vi "Toggle Allow Undefined Strings.vi"(8 "error in (no error)":errorcluster, 10 "Allow Undefined Strings":bool, 11 "List Data Type in":refnum<class "List Data Type.lvclass">) -> (0 "error out":errorcluster, 3 "List Data Type out":refnum<class "List Data Type.lvclass">)   [LabVIEW 2018, in "List Data Type.lvclass"]
uses:
  List Data Type.lvclass
  List Data Type.lvclass/List Data Type.ctl
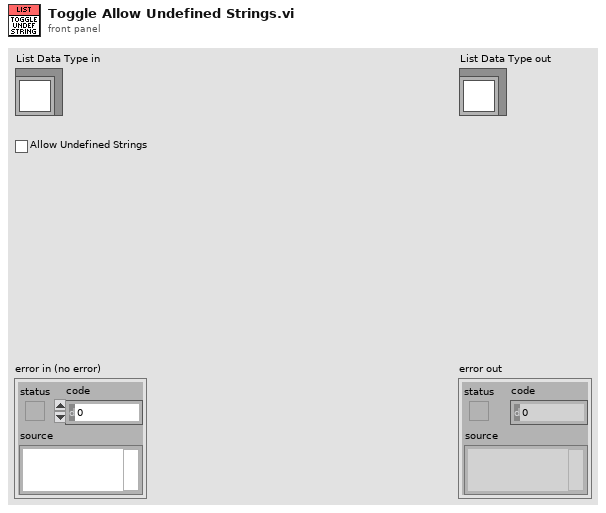
[diagram p1: front panel]
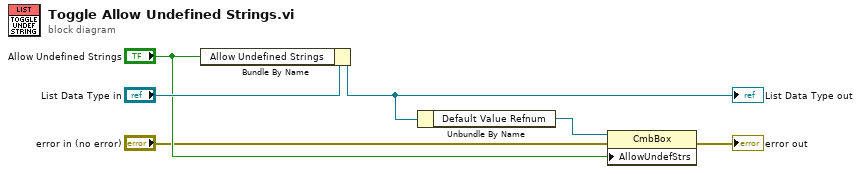
[diagram p0: block diagram]
diagram:
  n1 = Bundle By Name(cluster="List Data Type in", "Allow Undefined Strings"="Allow Undefined Strings") -> (w4:refnum<class "List Data Type.lvclass">)
  "List Data Type out" <- w4
  n2 = Unbundle By Name(w4) -> ("Default Value Refnum"=w2:refnum<vi>)
  n3 = property class="CmbBox"(reference=w2, error in="error in (no error)", "AllowUndefStrs"="Allow Undefined Strings") -> (error out=→"error out":errorcluster)  [unwired: 1 out]
